vi "Mover4_Control_Inverse_Kinematics_Stream_Conneciont_Kinect.vi"() -> ()   [LabVIEW 2015]
uses:
  <vilib>/Platform/TimedLoop/XDataNode/timing_clust.ctl
  <vilib>/Platform/TimedLoop/XDataNode/nitl_modes.ctl
  <vilib>/Platform/TimedLoop/XDataNode/wakeup.ctl
  <vilib>/Utility/miscctls.llb/LVRGBAColorTypeDef.ctl
  <vilib>/MakerHub/KinectOne/Private/Initialize Image [Color].vi
  Microsoft.Kinect
  C:/Program Files (x86)/National Instruments/LabVIEW 2015/vi.lib/MakerHub/KinectOne/Private/Libs/BodyFrameDataInterface.dll
  Program Files (x86)/National Instruments/LabVIEW 2015/vi.lib/MakerHub/KinectOne/Private/Libs/BodyFrameDataInterface.dll
  <vilib>/platform/TimedLoop/XDataNode/XDataNode.xnode
  <vilib>/robotics/Kinematics/Plotting/NI_Robotics_3DKinematics.lvlib
  <vilib>/MakerHub/KinectOne/KinectOne.lvlib
  <vilib>/Platform/TimedLoop/XDataNode/XDNodeRunTimeDep.lvlib
panel:
  out "Simulation":refnum<vi>(3d-picture)
  out "Motor positions (degree)":T1(array[cluster]) {"Error Code (bits)" format="%b"}
  out "stop button":bool
  out "Camera output":T2(plugin-control)
  out "Position Left Wrist (XYZ)":dbl[](array[numeric])
  in  "Reset To Zero?":bool
  out "Position not\nreachable?":bool=TRUE
  in  "Target IP Address":string="172.22.11.2"
  in  "Stop":bool
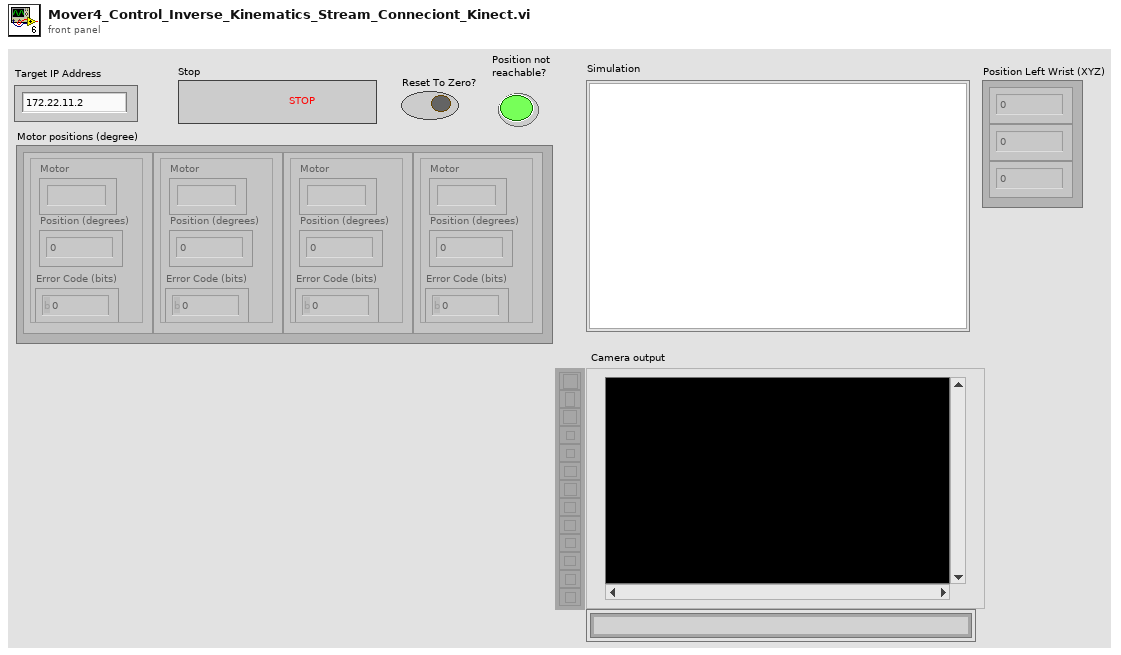
[diagram p1: front panel]
types:
  T1 = cluster{"Position (degrees)":i32, "Error Code (bits)":u8, "Motor":string}[]
  T2 = typedef "IMAQ Image.ctl" = refnum<image>
  T3 = typedef "LVRGBAColorTypeDef.ctl" = cluster{"Red":sgl, "Green":sgl, "Blue":sgl, "Alpha":sgl}
  T4 = cluster{"Desired Position":u16, "Enable?":bool, "Reset?":bool}[]
  T5 = cluster{"ID":u8, "Position":u16, "Error Code":u8}[]
  T6 = cluster{"Read Access":enum8{"Allowed", "Required", "None"}, "Write Access":enum8{"Allowed", "Required", "None"}}
  T7 = typedef "KinectOne.lvlib/KinectSensor References.ctl" = cluster{"KinectSensor":refnum<k24>, "MultiSourceFrameReader":refnum<k24>, "BodyFrameDataInterface":refnum<k24>}
  T8 = typedef "XDNodeRunTimeDep.lvlib/timing_clust.ctl" = cluster{"Expected End [f-1]":u64, "Actual End [f-1]":u64, "Finished Late? [f-1]":bool, "Expected End [i-1]":u64, "Actual End [i-1]":u64, "Finished Late? [i-1]":bool, "Expected Start [i]":u64, "Actual Start [i]":u64, "Expected Start [f]":u64, "Actual Start [f]":u64, "Source Name":string, "Structure Name":string, "Period":i64, "Deadline":i64, "Offset":i64, "Start":i64, "Priority":i32, "Timeout":i32, "Mode":T9, "Wakeup Reason":T10, "Error":errorcluster, "Source Type":string, "Secondary Source Type":string, "Global End Time":u64, "Global Start Time":u64, "Frame Duration":u64, "Iteration Duration":u64, "Assigned CPU":i32, "I/O Scan Engine Mode":u32}
  T9 = typedef "XDNodeRunTimeDep.lvlib/nitl_modes.ctl" = enum32{"No Change", "Process missed periods, maintain original phase", "Discard missed periods, maintain original phase", "Process missed periods, ignore original phase", "Discard missed periods, ignore original phase"}
  T10 = typedef "XDNodeRunTimeDep.lvlib/wakeup.ctl" = enum32{"Normal", "Aborted", "Asynchronous wakeup", "Timing source error", "Timed loop error", "Timeout"}
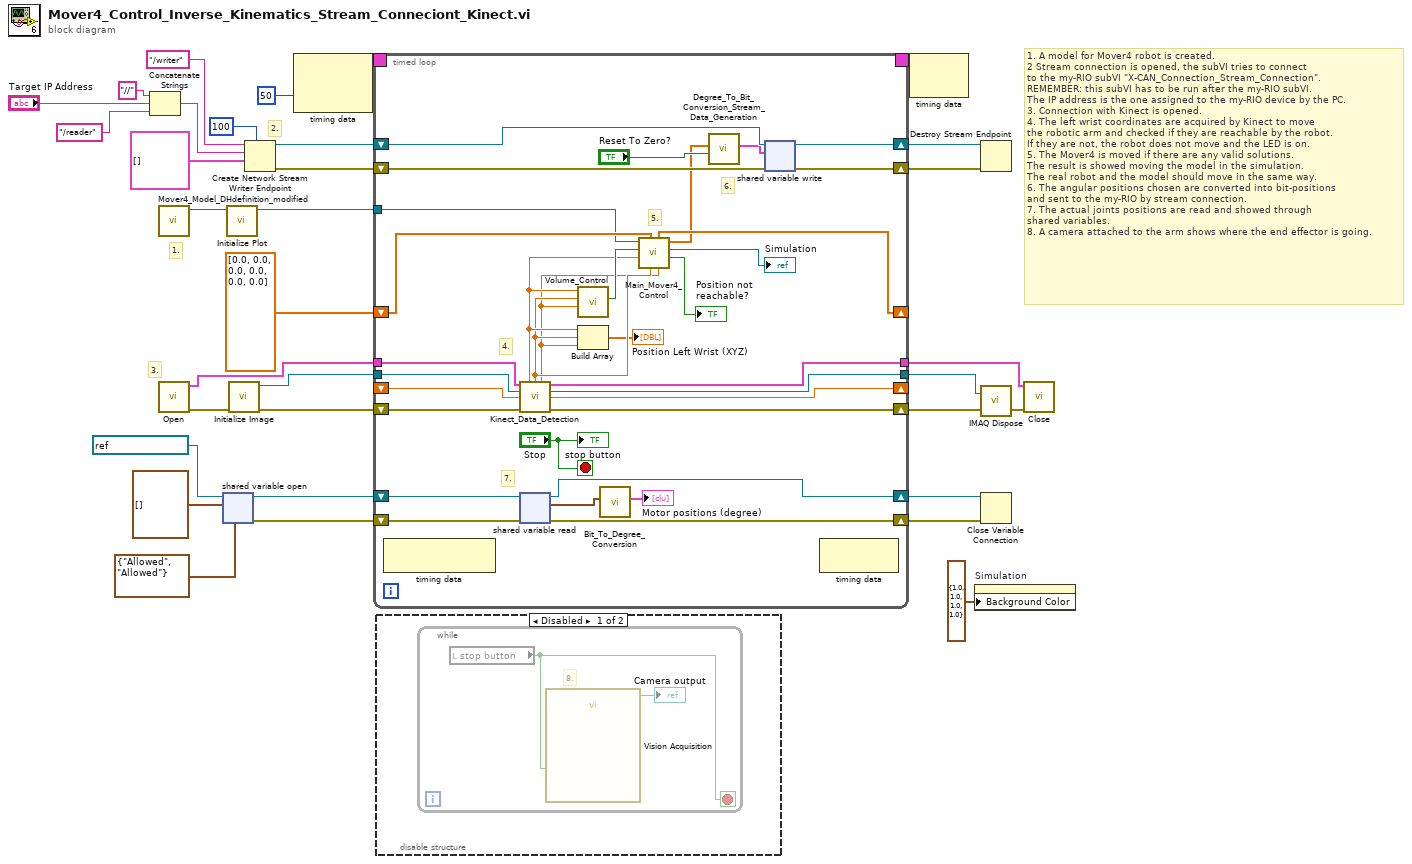
[diagram p0: block diagram]
diagram:
  # "3."
  # "2."
  # "1."
  # "1. A model for Mover4 robot is created.\n2 Stream connection is opened, the subVI tries to connect\nto the my-RIO subVI \"X-CAN_Connection_Stream_Connection\".\nREMEMBER: this subVI has to be run after the my-RIO subVI. \nThe IP address is the one assigned to the my-RIO device by the PC.\n3. Connection with Kinect is opened.\n4. The left wrist coordinates are acquired by Kinect to move \nthe robotic arm and checked if they are reachable by the robot.\nIf they are not, the robot does not move and the LED is on.\n5. The Mover4 is moved if there are any valid solutions.\nThe result is showed moving the model in the simulation. \nThe real robot and the model should move in the same way.\n6. The angular positions chosen are converted into bit-positions\nand sent to the my-RIO by stream connection.\n7. The actual joints positions are read and showed through\nshared variables.\n8. A camera attached to the arm shows where the end effector is going."
  n1 = Concatenate Strings("//", "Target IP Address", "/reader") -> (w26:string)
  n2 = call "Mover4_Model_DHdefinition_modified.vi"() -> ("serial arm out"=w13:refnum<class "NI_Robotics_6R Type 1 Serial Arm Class.lvclass">)  [unwired: 10 in, 1 out]
  n3 = call <vilib>:"Open.vi"() -> ("Error Out"=w12:errorcluster, "KinectSensor References out"=w11:T7)  [unwired: 10 in]
  n4 = shared-variable-open(refnum<k21> "ni.var.psp://stratom-myrio/Shared_Variables/New position" ("shared variable refnum in"), T5 [] ("New position 2"), T6 {"Read Access"=enum."Allowed", "Write Access"=enum."Allowed"} ("access")) -> (w33:refnum<k21>, w32:errorcluster)  [unwired: 1 in]
  n5 = call <vilib>:"Initialize Plot.vi"("serial arm in"=w13) -> ("serial arm out"=w14:refnum<class "NI_Robotics_6R Type 1 Serial Arm Class.lvclass">)  [unwired: 9 in, 1 out]
  n6 = call-poly <vilib>:"Initialize Image.vi"("Error In"=w12) -> ("Error Out"=w10:errorcluster, "Color Image"=w9:T2)  [unwired: 9 in]
  n7 = Create Network Stream Writer Endpoint(7:100 ("writer buffer size"), 9:T4 [] ("Commands 2"), 10:w26, 11:"/writer" ("reader name")) -> (0:w19:errorcluster, 3:w20:refnum<k21>)  [unwired: 3 in]
  n8 = node-c288(i64 50 ("Period")) -> (w4:T8)  [unwired: 1 in]
  n9 = timed-loop {
    shift-right: [w63] -> w29
    shift-left: w33 -> [w65]
    shift-right: [w62] -> w28
    shift-left: w32 -> [w64]
    shift-right: [w59] -> w18
    shift-left: w20 -> [w61]
    shift-right: [w58] -> w17
    shift-left: w19 -> [w60]
    shift-right: [w51] -> _
    shift-left: dbl[] [0.0, 0.0, 0.0, 0.0, 0.0, 0.0] ("current joint positions") -> [w54]
    tunnel: w14 -> [w53]
    tunnel: w11 -> [w49]
    tunnel: w9 -> [w48]
    shift-right: [w44] -> w7
    shift-left: w10 -> [w47]
    tunnel: [w46] -> w6
    tunnel: [w45] -> w5
    shift-right: [w38] -> _
    shift-left: _ -> [w39]
    timing: w4 -> [_]
    timing-out: [_] -> w3
    stop <- "Stop" stop-if-true
    # "7."
    # "6."
    # "5."
    # "4."
    n10 = node-c288() -> ()  [unwired: 1 in, 1 out]
    n11 = call "Kinect_Data_Detection.vi"("KinectSensor References in"=w49, "Image"=w48, "Distance from Kinect (m)"=w39, "error in (no error)"=w47) -> ("X (m)"=w43:dbl, "Y (m)"=w42:dbl, "Z (m)"=w41:dbl, "KinectSensor References"=w45:T7, "Image Out"=w46:T2, "Distance from Kinect (calibrated, m)"=w38:dbl, "Error Out"=w44:errorcluster)  [unwired: 5 in]
    n12 = shared-variable-read(w65, w64) -> (w63:refnum<k21>, w62:errorcluster, w36:T5)  [unwired: 1 out]
    n13 = call "Volume_Control.vi"("z (m)"=w41, "y (m)"=w42, "x (m)"=w43) -> ("Range acceptable?"=w56:bool)  [unwired: 8 in]
    n14 = Build Array(w43, w42, w41) -> (→"Position Left Wrist (XYZ)":dbl[])
    n15 = call "Bit_To_Degree_Conversion.vi"("Actual joints positions"=w36) -> ("Motor positions (degree)"=→"Motor positions (degree)":T1)  [unwired: 10 in]
    n16 = call "Main_Mover4_Control.vi"("Z (m)"=w41, "Y (m)"=w42, "current joint positions in"=w54, "X (m)"=w43, "Range acceptable?"=w56, "NI_Robotics_6R Type 1 Serial Arm Class in"=w53) -> ("Position not reachable?"=→"Position not\nreachable?":bool, "Simulation"=→"Simulation":refnum<vi>, "current joint positions degree"=w50:dbl[], "current joint positions out"=w51:dbl[])  [unwired: 2 in]
    n17 = call "Degree_To_Bit_Conversion_Stream_Data_Generation.vi"("Reset To Zero?"="Reset To Zero?", "Degree"=w50) -> ("Commands"=w57:T4)  [unwired: 9 in]
    n18 = shared-variable-write(w61, w60, w57) -> (w59:refnum<k21>, w58:errorcluster)  [unwired: 1 in, 1 out]
    n19 = node-c288() -> ()  [unwired: 1 in, 1 out]
    "stop button" <- "Stop"
  }
  n20 = disable-structure shown="Disabled" {
    frame Disabled {
      n21 = while {
        stop <- w68 stop-if-true
        # "8."
        n22 = local read "stop button"() -> (w68:bool)
        n23 = call "Vision Acquisition"("Stop (F)"=w68) -> ("Image Out"=→"Camera output":T2)  [unwired: 24 in, 2 out]
      }
    }
    frame Enabled {
    }
  }
  n24 = node-c288(w3) -> ()  [unwired: 1 out]
  n25 = property on="Simulation" class="SceneGraphDisp (strict)"("Background Color"=T3 {"Red"=1.0, "Green"=1.0, "Blue"=1.0, "Alpha"=1.0}) -> ()  [unwired: 2 in, 2 out]
  n26 = Destroy Stream Endpoint(8:w17, 11:w18) -> ()  [unwired: 1 out]
  n27 = call "IMAQ Dispose"("Image"=w6, "error in (no error)"=w7) -> ("error out"=w8:errorcluster)  [unwired: 4 in]
  n28 = Close Variable Connection(8:w28, 11:w29) -> ()  [unwired: 1 out]
  n29 = call <vilib>:"Close.vi"("Error In"=w8, "KinectSensor References"=w5) -> ()  [unwired: 9 in, 1 out]
